vi "UI Stop.vi"() -> ()   [LabVIEW 2014]
panel:
  in  "UI STOP":bool
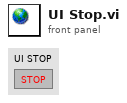
[diagram p1: front panel]
diagram:
